vi "Autonomous Independent.vi"() -> ()   [LabVIEW 2011]
doc: "This VI is called when autonomous begins, and will automatically be terminated when autonomous ends. You can carry out timed or sensor driven robot movement independently without needing to return to the caller."
uses:
  Robot Global Data.vi
panel:
  in  "EncoderDistance":dbl
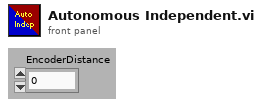
[diagram p1: front panel]
types:
  T1 = typedef "WPI_MotorControlDeviceRef.ctl" = cluster{"DeviceStatus":errorcluster, "Type":enum16{"PWM", "CAN"}, "PWM":cluster{"Digital Module":T2, "PWM Channel":T3, "DeadBand":T4}, "CAN":cluster{"Device Number":u8, "Control Mode":T5, "Semaphore":T6, "Max Vout":dbl}, "Invert":bool, "TransformRef":T7, "InvTransformRef":T7}
  T2 = typedef "FPGA_TypedefDigitalModule.ctl" = enum16{"Digital Module 1", "Digital Module 2"}
  T3 = typedef "FPGA_DIOPWMChannel.ctl" = enum8{"PWM 1", "PWM 2", "PWM 3", "PWM 4", "PWM 5", "PWM 6", "PWM 7", "PWM 8", "PWM 9", "PWM 10", "Invalid"}
  T4 = typedef "WPI_PWMDeadband.ctl" = cluster{"Name":string, "maxPositivePwm":i32, "minPositivePwm":i32, "centerPwm":i32, "maxNegativePwm":i32, "minNegativePwm":i32, "angularRange":u16}
  T5 = typedef "WPI_CANJaguar_ControlMode.ctl" = enum8{"Percent VBus", "Current", "Speed", "Position", "Voltage"}
  T6 = typedef "Semaphore RefNum" = refnum<k1>
  T7 = typedef "WPI_PWMTransform_ConPane.ctl" = refnum<vi>
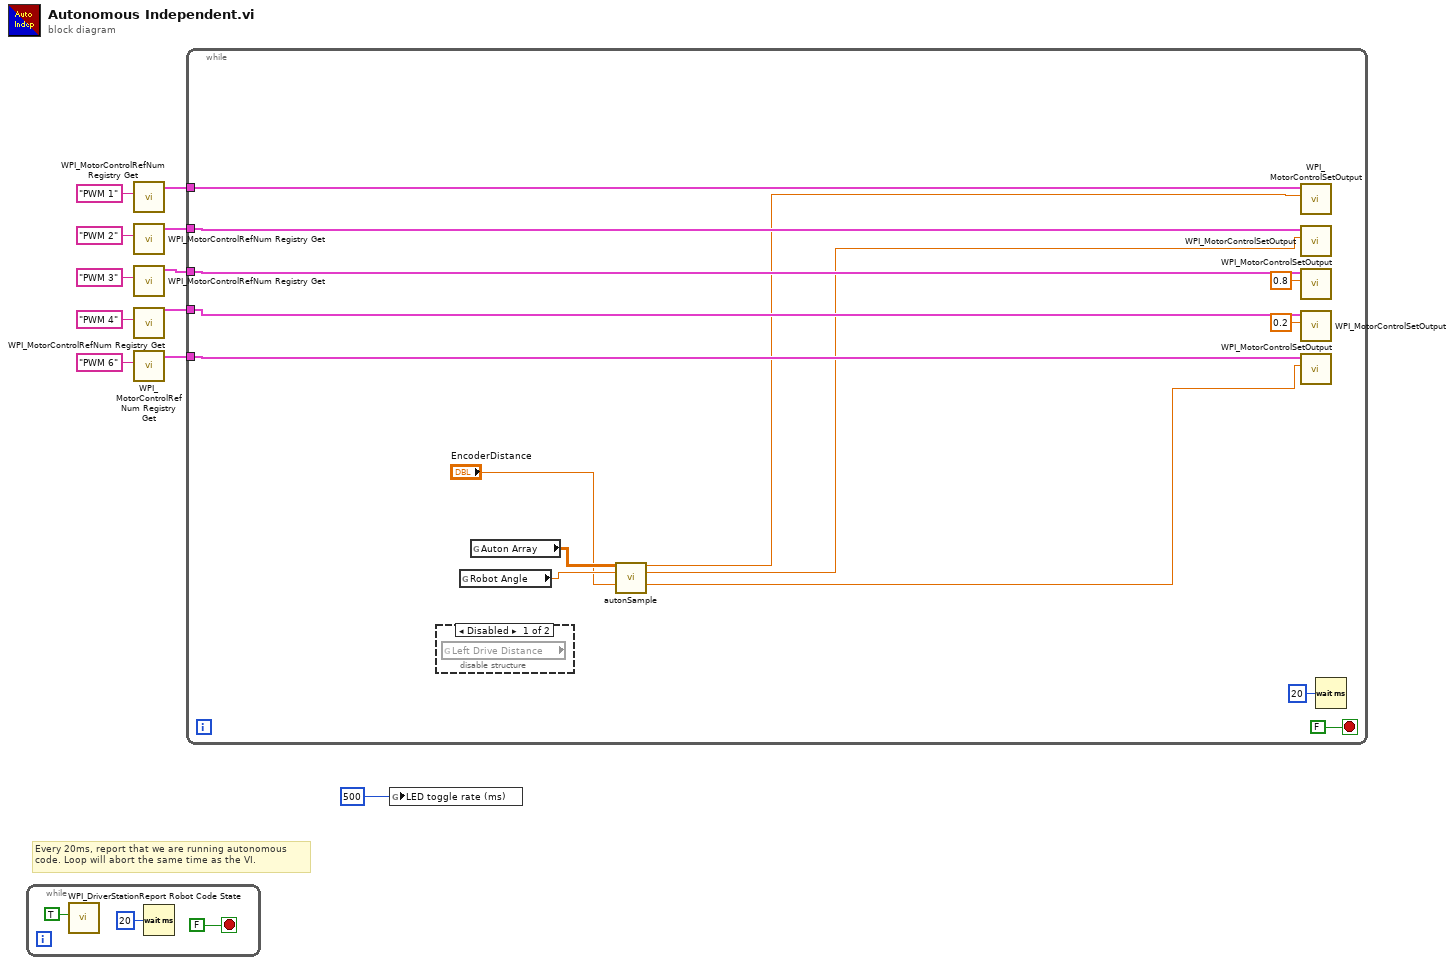
[diagram p0: block diagram]
diagram:
  # "Every 20ms, report that we are running autonomous\ncode. Loop will abort the same time as the VI."
  n1 = while {
    stop <- FALSE stop-if-true
    n2 = call <vilib>:"WPI_DriverStationReport Robot Code State.vi"("Autonomous"=TRUE) -> ()  [unwired: 10 in, 1 out]
    n3 = Wait (ms)(milliseconds to wait=u32 20) -> ()  [unwired: 1 out]
  }
  n4 = call <vilib>:"WPI_MotorControlRefNum Registry Get.vi"("refnum name"="PWM 1") -> ("MotorControlDevRef"=w5:T1)  [unwired: 9 in, 1 out]
  n5 = call <vilib>:"WPI_MotorControlRefNum Registry Get.vi"("refnum name"="PWM 2") -> ("MotorControlDevRef"=w4:T1)  [unwired: 9 in, 1 out]
  n6 = call <vilib>:"WPI_MotorControlRefNum Registry Get.vi"("refnum name"="PWM 3") -> ("MotorControlDevRef"=w3:T1)  [unwired: 9 in, 1 out]
  n7 = call <vilib>:"WPI_MotorControlRefNum Registry Get.vi"("refnum name"="PWM 4") -> ("MotorControlDevRef"=w2:T1)  [unwired: 9 in, 1 out]
  n8 = call <vilib>:"WPI_MotorControlRefNum Registry Get.vi"("refnum name"="PWM 6") -> ("MotorControlDevRef"=w1:T1)  [unwired: 9 in, 1 out]
  n9 = while {
    tunnel: w5 -> [w27]
    tunnel: w4 -> [w26]
    tunnel: w3 -> [w25]
    tunnel: w2 -> [w24]
    tunnel: w1 -> [w23]
    stop <- FALSE stop-if-true
    n10 = disable-structure shown="Disabled" {
      frame Disabled {
        n11 = global read "Robot Global Data.vi" "Left Drive Distance"() -> ()  [unwired: 1 out]
      }
      frame Enabled {
      }
    }
    n12 = global read "Robot Global Data.vi" "Robot Angle"() -> (w21:dbl)
    n13 = global read "Robot Global Data.vi" "Auton Array"() -> (w22:dbl[][])
    n14 = call "autonSample.vi"("Auton Array"=w22, "MeasuredHeading"=w21, "EncoderDistance"="EncoderDistance") -> ("Left Drive"=w20:dbl, "Right Drive"=w19:dbl, "Turret Rotation"=w16:dbl)  [unwired: 8 in, 2 out]
    n15 = call <vilib>:"WPI_MotorControlSetOutput.vi"("Output"=w20, "MotorControlDevRef"=w27) -> ()  [unwired: 8 in, 2 out]
    n16 = call <vilib>:"WPI_MotorControlSetOutput.vi"("Output"=w19, "MotorControlDevRef"=w26) -> ()  [unwired: 8 in, 2 out]
    n17 = call <vilib>:"WPI_MotorControlSetOutput.vi"("Output"=0.8, "MotorControlDevRef"=w25) -> ()  [unwired: 8 in, 2 out]
    n18 = call <vilib>:"WPI_MotorControlSetOutput.vi"("Output"=0.2, "MotorControlDevRef"=w24) -> ()  [unwired: 8 in, 2 out]
    n19 = call <vilib>:"WPI_MotorControlSetOutput.vi"("Output"=w16, "MotorControlDevRef"=w23) -> ()  [unwired: 8 in, 2 out]
    n20 = Wait (ms)(milliseconds to wait=u32 20) -> ()  [unwired: 1 out]
  }
  n21 = global write "Robot Global Data.vi" "LED toggle rate (ms)"(u32 500 ("LED ms toggle rate")) -> ()
